vi "Write Vertical Scrollbar.vi"(5 "Vertical Scrollbar":bool, 9 "String in":refnum<class "String.lvclass">) -> (3 "String out":refnum<class "String.lvclass">)   [LabVIEW 2014, in "String.lvclass"]
uses:
  String.lvclass
  String.lvclass/String.ctl
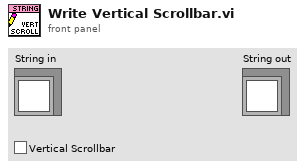
[diagram p1: front panel]
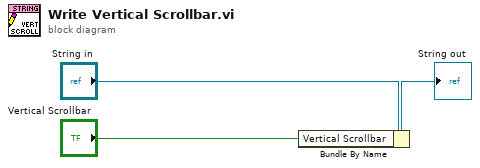
[diagram p0: block diagram]
diagram:
  n1 = Bundle By Name(cluster="String in", "Vertical Scrollbar"="Vertical Scrollbar") -> (→"String out":refnum<class "String.lvclass">)
